vi "Save Report.vi"(6 "In cluster":T1={"Pass/Fail"="PASS", "Cycle time"="67.86 s", "Model"="Y1k s", "Variant name"="Y1k_LO-MT-RHS-CNG-0N39", "Start time"="Y1k_LO-MT-RHS-CNG-0N39", "st"="PASS"}, 7 "Barcode":string, 8 "error in (no error)":errorcluster, 9 "ItemNames":string[][](array[string]), 10 "Log Report":bool, 11 "Report path":path) -> (0 "error out":errorcluster)   [LabVIEW 2017]
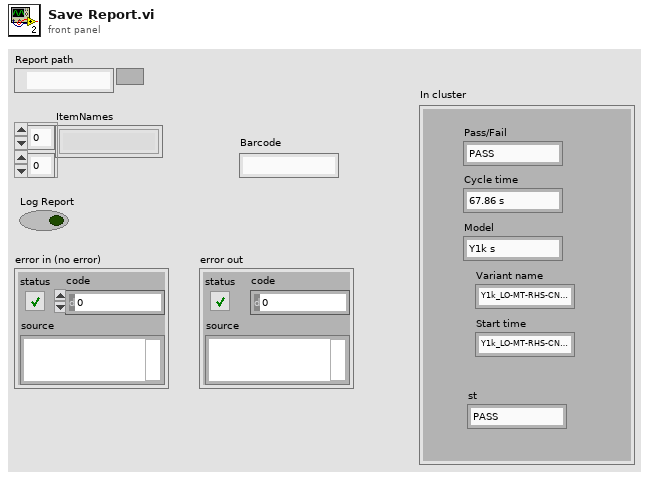
[diagram p1: front panel]
types:
  T1 = cluster{"Pass/Fail":string, "Cycle time":string, "Model":string, "Variant name":string, "Start time":string, "st":string}
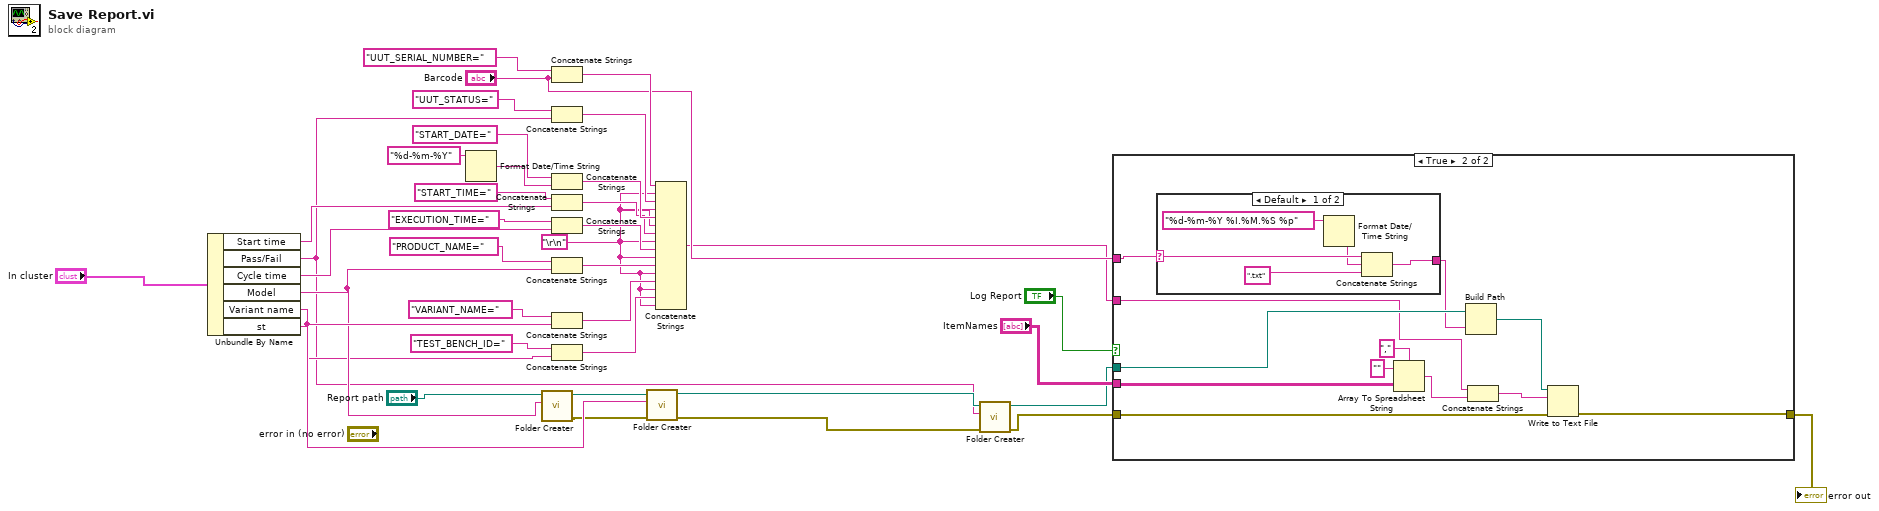
[diagram p0: block diagram]
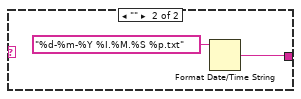
[diagram p3: hidden frame]
diagram:
  w13 = "\r\n"
  n1 = Unbundle By Name("In cluster") -> ("Start time"=w12:string, "Pass/Fail"=w1:string, "Cycle time"=w16:string, "Model"=w9:string, "Variant name"=w11:string, "st"=w2:string)
  n2 = Format Date/Time String(time format string (%c)="%d-%m-%Y") -> (date/time string=w19:string)  [unwired: 2 in]
  n3 = call "Folder Creater.vi"("Variant name"=w9, "dup path in"="Report path") -> ("error out"=w7:errorcluster, "dup path out"=w8:path)  [unwired: 8 in]
  n4 = Concatenate Strings("UUT_SERIAL_NUMBER=" ("string"), "Barcode") -> (w28:string)
  n5 = Concatenate Strings("UUT_STATUS=" ("string"), w1) -> (w27:string)
  n6 = Concatenate Strings("START_DATE=" ("string"), w19) -> (w26:string)
  n7 = Concatenate Strings("START_TIME=" ("string"), w12) -> (w14:string)
  n8 = Concatenate Strings("EXECUTION_TIME=" ("string"), w16) -> (w25:string)
  n9 = Concatenate Strings("PRODUCT_NAME=" ("string"), w9) -> (w24:string)
  n10 = Concatenate Strings("VARIANT_NAME=" ("string"), w11) -> (w23:string)
  n11 = Concatenate Strings("TEST_BENCH_ID=" ("string"), w2) -> (w22:string)
  n12 = call "Folder Creater.vi"("error in (no error)"=w7, "Variant name"=w11, "dup path in"=w8) -> ("error out"=w5:errorcluster, "dup path out"=w6:path)  [unwired: 7 in]
  n13 = Concatenate Strings(w28, w13, w27, w13, w26, w13, w14, w13, w25, w13, w24, w13, w23, w13, w22, w13) -> (w18:string)
  n14 = call "Folder Creater.vi"("error in (no error)"=w5, "Variant name"=w1, "dup path in"=w6) -> ("error out"=w3:errorcluster, "dup path out"=w4:path)  [unwired: 7 in]
  n15 = case shown="True" "Log Report" {
    tunnel: w4 -> [_ w46]
    tunnel: w3 -> [w39 w47]
    tunnel: [w39 w45] -> w37
    tunnel: "ItemNames" -> [_ w49]
    tunnel: "Barcode" -> [_ w43]
    tunnel: w18 -> [_ w40]
    frame False {
    }
    frame True {
      n16 = case shown="Default" w43 {
        selector: w43 -> [w56 _]
        tunnel: [w55 w58] -> w42
        frame Default {
          n17 = Format Date/Time String(time format string (%c)="%d-%m-%Y %I.%M.%S %p") -> (date/time string=w53:string)  [unwired: 2 in]
          n18 = Concatenate Strings(w56, w53, ".txt" ("string")) -> (w55:string)
        }
        frame "" {
          n19 = Format Date/Time String(time format string (%c)="%d-%m-%Y %I.%M.%S %p.txt") -> (date/time string=w58:string)  [unwired: 2 in]
        }
      }
      n20 = Array To Spreadsheet String(delimiter (Tab)=",", array=w49, 3:"" ("format string")) -> (spreadsheet string=w48:string)
      n21 = Build Path(base path=w46, name or relative path=w42) -> (appended path=w44:path)
      n22 = Concatenate Strings(w40, w48) -> (w41:string)
      n23 = Write to Text File(file (use dialog)=w44, text=w41, error in=w47) -> (error out=w45:errorcluster)  [unwired: 1 in, 2 out]
    }
  }
  "error out" <- w37
